vi "Untitled 4.vi"   [LabVIEW 2016]
uses:
  <vilib>/DAQmx/write.llb/DAQmx Write.vi
  <vilib>/DAQmx/write.llb/DAQmx Write (Digital 1D Wfm NChan NSamp).vi
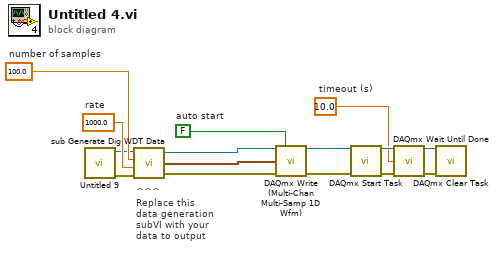
[diagram p0: block diagram]
diagram:
  w3 = 10.0  # timeout (s)
  w11 = 1000.0  # rate
  w12 = 100.0  # number of samples
  w15 = FALSE  # auto start
  # "^^^\nReplace this\ndata generation\nsubVI with your\ndata to output"
  n1 = call "Untitled 9"() -> ("error out"=w1:errorcluster, "task out"=w2:refnum<k21>)  [unwired: 10 in]
  n2 = call <vilib>:"sub Generate Dig WDT Data.vi"("task in"=w2, "number of samples"=w12, "update rate"=w11, "error in"=w1) -> ("task out"=w13:refnum<k21>, "data"=w4:digitalwaveform[], "error out"=w14:errorcluster)  [unwired: 1 in]
  n3 = call-poly "DAQmx Write (Multi-Chan Multi-Samp 1D Wfm).vi"("task/channels in"=w13, "auto start"=w15, "data"=w4, "error in"=w14) -> ("task out"=w7:refnum<k21>, "error out"=w6:errorcluster)  [unwired: 9 in, 1 out]
  n4 = call <vilib>:"DAQmx Start Task.vi"("task/channels in"=w7, "error in"=w6) -> ("task out"=w10:refnum<k21>, "error out"=w9:errorcluster)  [unwired: 12 in]
  n5 = call <vilib>:"DAQmx Wait Until Done.vi"("task/channels in"=w10, "timeout (sec)"=w3, "error in"=w9) -> ("task out"=w5:refnum<k21>, "error out"=w8:errorcluster)  [unwired: 11 in]
  n6 = call <vilib>:"DAQmx Clear Task.vi"("task in"=w5, "error in"=w8) -> ()  [unwired: 13 in, 1 out]
